vi "GetClass.vi"(5 "name":string, 6 "error in":errorcluster, 9 "PythonConverter_BD in":refnum<class "PyConvBD.lvclass">) -> (0 "error out":errorcluster, 3 "PythonConverter_BD out":refnum<class "PyConvBD.lvclass">, 4 "class":string)   [LabVIEW 2014, in "Raspberry Pi Compatible Compiler for LabVIEW.lvlib" / "PyConvBD.lvclass"]
uses:
  PyConvBD.lvclass
  PyConvBD.lvclass/PyConvBD.ctl
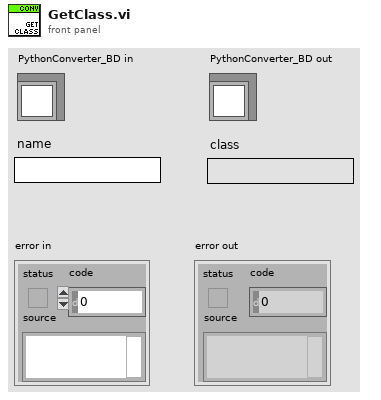
[diagram p1: front panel]
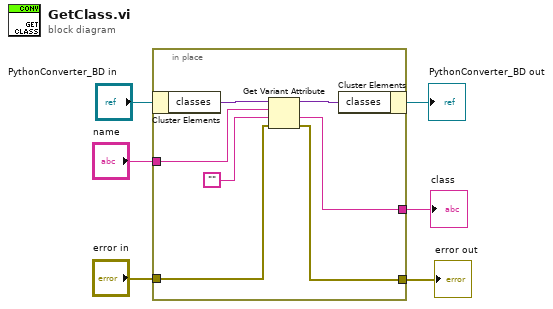
[diagram p0: block diagram]
diagram:
  n1 = in-place {
    in-place-border: "error in" -> [w12]
    in-place-border: [w11] -> w3
    in-place-border: "name" -> [w10]
    in-place-border: [w7] -> w1
    n2 = in-place-cluster #1("PythonConverter_BD in") -> ("classes"=w9:variant)
    n3 = Get Variant Attribute(Variant=w9, name=w10, default value (empty Variant)="", error in=w12) -> (duplicate Variant=w13:variant, value=w7:string, error out=w11:errorcluster)  [unwired: 1 out]
    n4 = in-place-cluster #1("classes"=w13) -> (→"PythonConverter_BD out":refnum<class "PyConvBD.lvclass">)
  }
  "error out" <- w3
  "class" <- w1
